vi "absMove.vi"(0 "CurrentX引用":refnum<vi>, 1 "CurrentY引用":refnum<vi>, 2 "TargetX":dbl, 3 "TargetY":dbl, 4 "Param_StepDis":dbl, 5 "错误输入（无错误）":errorcluster, 6 "模式":enum16{"快速移动", "规划速度"}(ring)) -> (19 "错误输出":errorcluster)   [LabVIEW 2011]
uses:
  API/API DYM.lvlib
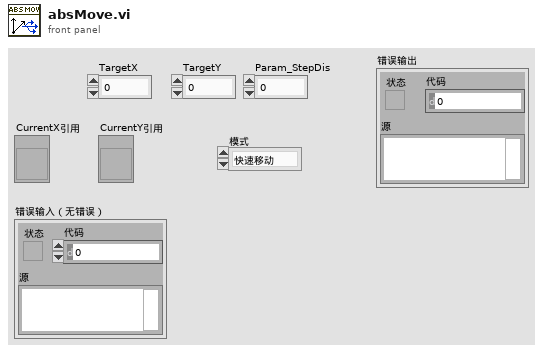
[diagram p1: front panel]
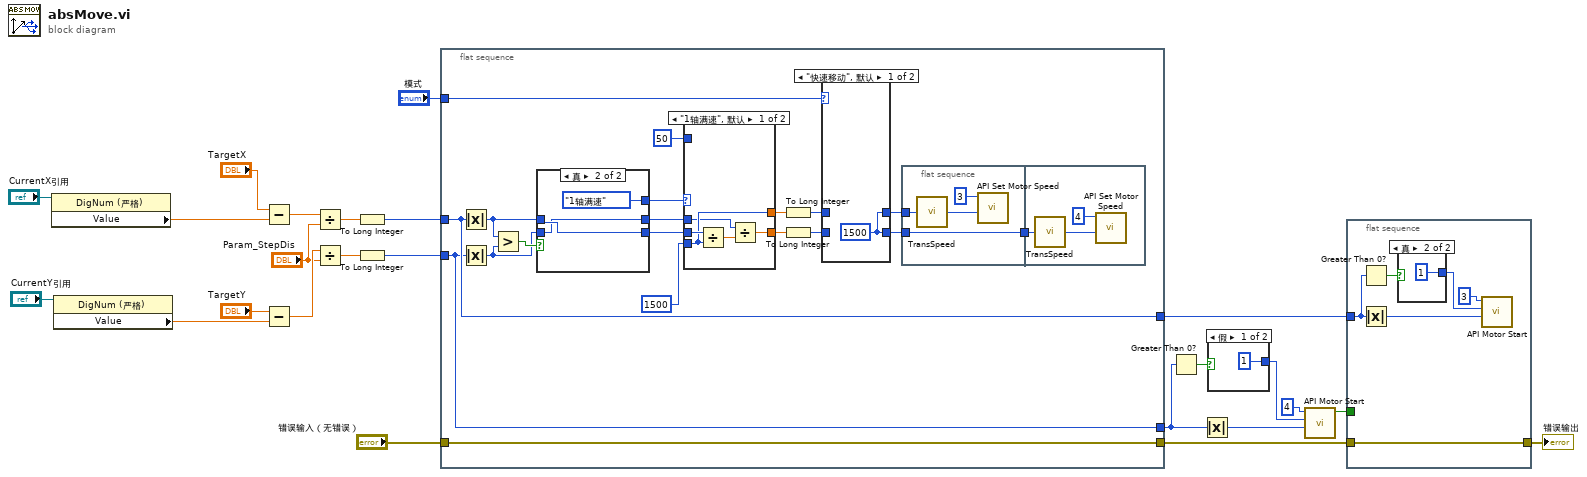
[diagram p0: block diagram]
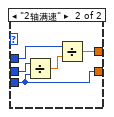
[diagram p3: hidden frame]
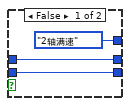
[diagram p4: hidden frame]
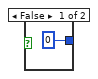
[diagram p5: hidden frame]
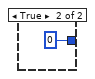
[diagram p6: hidden frame]
diagram:
  n1 = property class="DigNum (严格)"(reference="CurrentX引用") -> ("Value"=w4:dbl)  [unwired: 1 in, 2 out]
  n2 = property class="DigNum (严格)"(reference="CurrentY引用") -> ("Value"=w3:dbl)  [unwired: 1 in, 2 out]
  n3 = Subtract(x="TargetX", y=w4) -> (x-y=w22:dbl)
  n4 = Subtract(x="TargetY", y=w3) -> (x-y=w21:dbl)
  n5 = Divide(x=w22, y="Param_StepDis") -> (x/y=w14:dbl)
  n6 = Divide(x=w21, y="Param_StepDis") -> (x/y=w19:dbl)
  n7 = To Long Integer(number=w14) -> (32bit integer=w13:i32)
  n8 = To Long Integer(number=w19) -> (32bit integer=w11:i32)
  n9 = flat-sequence {
    tunnel: w13 -> [w43]
    tunnel: [w43] -> w12
    tunnel: w11 -> [w42]
    tunnel: [w42] -> w10
    tunnel: "模式" -> [w31]
    tunnel: "错误输入（无错误）" -> [w25]
    tunnel: [w25] -> w6
    frame #0 {
      n10 = Absolute Value(x=w43) -> (abs(x)=w37:i32)
      n11 = Absolute Value(x=w42) -> (abs(x)=w36:i32)
      n12 = Greater?(x=w37, y=w36) -> (0:w41:bool)
      n13 = case shown="真" w41 {
        tunnel: [enum16{"1轴满速", "2轴满速"}."2轴满速" enum16{"1轴满速", "2轴满速"}."1轴满速"] -> w40
        tunnel: w37 -> [w65 w68]
        tunnel: w36 -> [w64 w67]
        tunnel: [w64 w68] -> w35
        tunnel: [w65 w67] -> w34
        frame False {
        }
        frame True {
        }
      }
      n14 = case shown="\"1轴满速\", 默认" w40 {
        tunnel: 1500 -> [w56 w62]
        tunnel: 50 -> [_ _]
        tunnel: w35 -> [w58 w63]
        tunnel: w34 -> [w55 w60]
        tunnel: [w56 w59] -> w32
        tunnel: [w54 w62] -> w33
        frame "1轴满速", Default {
          n15 = Divide(x=w58, y=w56) -> (x/y=w57:dbl)
          n16 = Divide(x=w55, y=w57) -> (x/y=w54:dbl)
        }
        frame "2轴满速" {
          n17 = Divide(x=w63, y=w62) -> (x/y=w61:dbl)
          n18 = Divide(x=w60, y=w61) -> (x/y=w59:dbl)
        }
      }
      n19 = To Long Integer(number=w32) -> (32bit integer=w30:i32)
      n20 = To Long Integer(number=w33) -> (32bit integer=w29:i32)
      n21 = case shown="\"快速移动\", 默认" w31 {
        tunnel: w30 -> [_ w46]
        tunnel: [w44 w46] -> w28
        tunnel: [w44 w45] -> w27
        tunnel: w29 -> [_ w45]
        frame "快速移动", Default {
          w44 = 1500
        }
        frame "规划速度" {
        }
      }
      n22 = flat-sequence {
        tunnel: w28 -> [w48]
        tunnel: w27 -> [w49]
        tunnel: [w49] -> w26
        tunnel: w26 -> [w52]
        frame #0 {
          n23 = call "TransSpeed.vi"("Speed_In"=w48) -> ("Speed_Out"=w47:i32)
          n24 = call "API Set Motor Speed.vi"("motorSpeed"=w47, "motorNum"=3) -> ()  [unwired: 9 in, 1 out]
        }
        frame #1 {
          n25 = call "TransSpeed.vi"("Speed_In"=w52) -> ("Speed_Out"=w51:i32)
          n26 = call "API Set Motor Speed.vi"("motorSpeed"=w51, "motorNum"=4) -> ()  [unwired: 9 in, 1 out]
        }
      }
    }
  }
  n27 = Greater Than 0?(x=w10) -> (x > 0?=w18:bool)
  n28 = Absolute Value(x=w10) -> (abs(x)=w9:i32)
  n29 = case shown="假" w18 {
    tunnel: [1 0] -> w17
    frame False {
    }
    frame True {
    }
  }
  n30 = call "API Motor Start.vi"("stepNum"=w9, "direction"=w17, "motorNum"=4) -> ("motorStart return value"=w16:bool)  [unwired: 8 in]
  n31 = flat-sequence {
    tunnel: w16 -> [_]
    tunnel: w12 -> [w74]
    tunnel: w6 -> [w72]
    tunnel: [w72] -> w5
    frame #0 {
      n32 = Greater Than 0?(x=w74) -> (x > 0?=w77:bool)
      n33 = Absolute Value(x=w74) -> (abs(x)=w73:i32)
      n34 = case shown="真" w77 {
        tunnel: [0 1] -> w76
        frame False {
        }
        frame True {
        }
      }
      n35 = call "API Motor Start.vi"("stepNum"=w73, "direction"=w76, "motorNum"=3) -> ()  [unwired: 8 in, 1 out]
    }
  }
  "错误输出" <- w5
